vi "add_AccelWithCovarianceStamped.vi"(6 "AccelCovariance":T1={"Vector"={"Linear"={"x"=0.0, "y"=0.0, "z"=0.0}, "Angular"={"x"=0.0, "y"=0.0, "z"=0.0}}, "Covariance"=[0.0, 0.0, 0.0, 0.0, 0.0]}, 7 "msg in":string) -> (3 "msg out":string)   [LabVIEW 2012]
doc: "Flattens a stamped acceleration with covariance into a message"
panel:
  in  "Stamp":cluster{"frame_id":string, "reset seq?":bool}
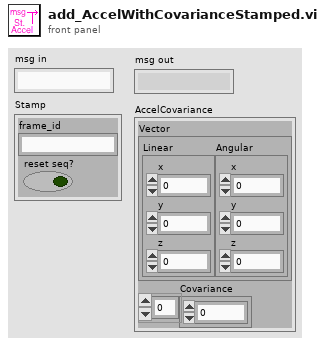
[diagram p1: front panel]
types:
  T1 = cluster{"Vector":cluster{"Linear":cluster{"x":dbl, "y":dbl, "z":dbl}, "Angular":cluster{"x":dbl, "y":dbl, "z":dbl}}, "Covariance":dbl[]}
  T2 = cluster{"Linear":cluster{"x":dbl, "y":dbl, "z":dbl}, "Angular":cluster{"x":dbl, "y":dbl, "z":dbl}}
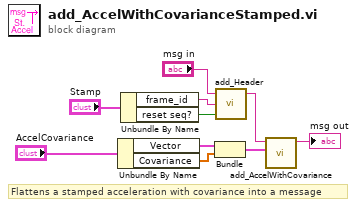
[diagram p0: block diagram]
diagram:
  # "Flattens a stamped acceleration with covariance into a message"
  n1 = Unbundle By Name("AccelCovariance") -> ("Vector"=w7:T2, "Covariance"=w6:dbl[])
  n2 = Unbundle By Name("Stamp") -> ("frame_id"=w2:string, "reset seq?"=w1:bool)
  n3 = Bundle("Vector"=w7, "Covariance"=w6) -> (w5:T1)  [unwired: 1 in]
  n4 = call "add_Header.vi"("reset seq?"=w1, "frame_id"=w2, "msg in"="msg in") -> ("msg out"=w4:string)  [unwired: 2 in]
  n5 = call "add_AccelWithCovariance.vi"("AccelCovariance"=w5, "msg in"=w4) -> ("msg out"=→"msg out":string)  [unwired: 5 in]
